vi "GetProperties.vi"(8 "error in":errorcluster, 11 "String in":refnum<class "String.lvclass">) -> (0 "error out":errorcluster, 3 "String out":refnum<class "String.lvclass">)   [LabVIEW 2014, in "String.lvclass"]
uses:
  String.lvclass
  String.lvclass/String.ctl
  Control/Control.lvclass
  Text/Text.lvclass
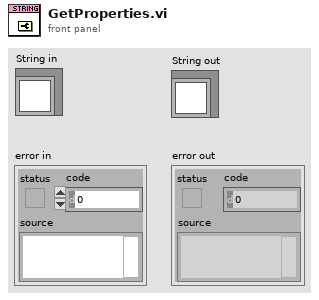
[diagram p1: front panel]
types:
  T1 = typedef "LVBoundsTypeDef.ctl" = cluster{"Width":u32, "Height":u32}
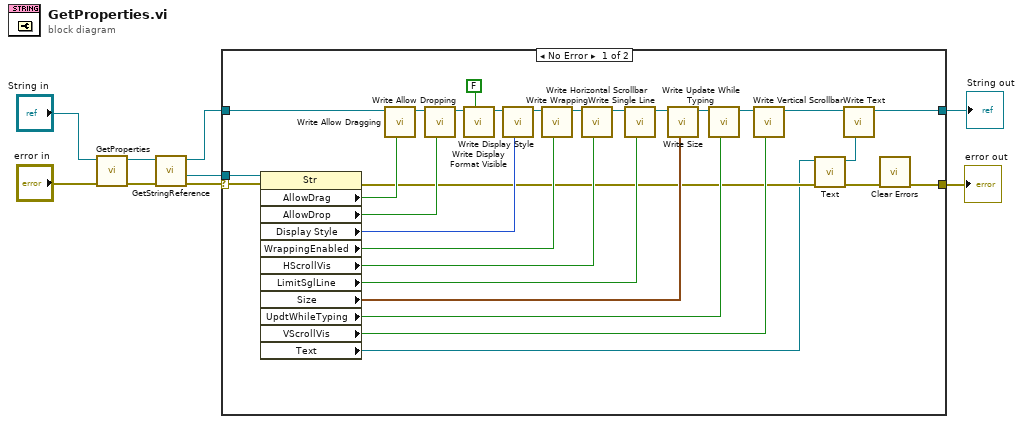
[diagram p0: block diagram]
diagram:
  n1 = call-parent "GetProperties.vi"("error in"="error in", "Control in"="String in") -> ("error out"=w6:errorcluster, "Control out"=w7:refnum<class "String.lvclass">)  [unwired: 8 in]
  n2 = call "GetStringReference.vi"("error in"=w6, "String in"=w7) -> ("error out"=w5:errorcluster, "String reference"=w4:refnum<vi>, "String out"=w3:refnum<class "String.lvclass">)  [unwired: 7 in]
  n3 = case shown="No Error" w5 {
    selector: w5 -> [w37 w39]
    tunnel: w4 -> [w38 _]
    tunnel: w3 -> [w36 w40]
    tunnel: [w13 w40] -> w1
    tunnel: [w10 w39] -> w2
    frame No Error {
      n4 = property on="Property Node" class="Str"(reference=w38, error in=w37) -> (error out=w17:errorcluster, "AllowDrag"=w35:bool, "AllowDrop"=w33:bool, "Display Style"=w30:u32, "WrappingEnabled"=w28:bool, "HScrollVis"=w26:bool, "LimitSglLine"=w24:bool, "Size"=w22:T1, "UpdtWhileTyping"=w20:bool, "VScrollVis"=w18:bool, "Text"=w16:refnum<vi>)  [unwired: 1 out]
      n5 = call "Write Allow Dragging.vi"("Allow Dragging"=w35, "String in"=w36) -> ("String out"=w34:refnum<class "String.lvclass">)  [unwired: 7 in]
      n6 = call "Write Allow Dropping.vi"("Allow Dropping"=w33, "String in"=w34) -> ("String out"=w32:refnum<class "String.lvclass">)  [unwired: 7 in]
      n7 = call "Write Display Format Visible.vi"("Display Format Visible"=FALSE, "String in"=w32) -> ("String out"=w31:refnum<class "String.lvclass">)  [unwired: 7 in]
      n8 = call "Write Display Style.vi"("Display Style"=w30, "String in"=w31) -> ("String out"=w29:refnum<class "String.lvclass">)  [unwired: 7 in]
      n9 = call "Write Wrapping.vi"("Wrapping"=w28, "String in"=w29) -> ("String out"=w27:refnum<class "String.lvclass">)  [unwired: 7 in]
      n10 = call "Write Horizontal Scrollbar.vi"("Horizontal Scrollbar"=w26, "String in"=w27) -> ("String out"=w25:refnum<class "String.lvclass">)  [unwired: 7 in]
      n11 = call "Write Single Line.vi"("Single Line"=w24, "String in"=w25) -> ("String out"=w23:refnum<class "String.lvclass">)  [unwired: 7 in]
      n12 = call "Write Size.vi"("Size"=w22, "String in"=w23) -> ("String out"=w21:refnum<class "String.lvclass">)  [unwired: 7 in]
      n13 = call "Write Update While Typing.vi"("Update While Typing"=w20, "String in"=w21) -> ("String out"=w19:refnum<class "String.lvclass">)  [unwired: 7 in]
      n14 = call "Write Vertical Scrollbar.vi"("Vertical Scrollbar"=w18, "String in"=w19) -> ("String out"=w15:refnum<class "String.lvclass">)  [unwired: 7 in]
      n15 = call "Text.vi"("error in"=w17, "GObj Refnum"=w16) -> ("error out"=w12:errorcluster, "Text out"=w14:refnum<class "Text.lvclass">)  [unwired: 8 in]
      n16 = call "Write Text.vi"("Text"=w14, "String in"=w15) -> ("String out"=w13:refnum<class "String.lvclass">)  [unwired: 7 in]
      n17 = call <vilib>:"Clear Errors.vi"("error in (no error)"=w12) -> ("error out"=w10:errorcluster)  [unwired: 5 in, 1 out]
    }
    frame Error {
    }
  }
  "error out" <- w2
  "String out" <- w1
